vi "sv_Check Tach Info.vi"(0 "tach info":T1 {"threshold [V]" format="%.2f"}) -> (4 "avg on n pulses":i32, 6 "pulse/revolution (1)":i32, 8 "threshold":dbl format="%.2f", 10 "pulse width":i32, 15 "error code":u32)   [LabVIEW 2017]
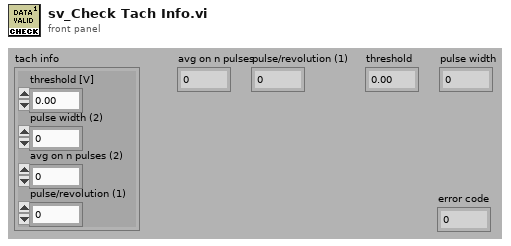
[diagram p1: front panel]
types:
  T1 = cluster{"threshold [V]":dbl, "pulse width (2)":i32, "avg on n pulses (2)":i32, "pulse/revolution (1)":i32}
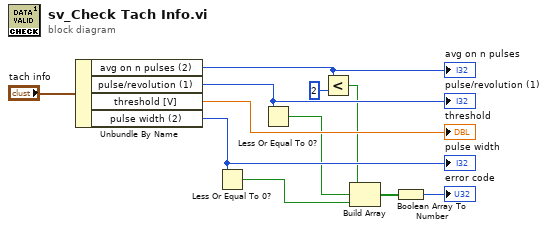
[diagram p0: block diagram]
diagram:
  n1 = Unbundle By Name("tach info") -> ("avg on n pulses (2)"=w6:i32, "pulse/revolution (1)"=w7:i32, "threshold [V]"=→"threshold":dbl, "pulse width (2)"=w10:i32)
  "pulse/revolution (1)" <- w7
  "avg on n pulses" <- w6
  "pulse width" <- w10
  n2 = Less Or Equal To 0?(x=w10) -> (x <= 0?=w3:bool)
  n3 = Less Or Equal To 0?(x=w7) -> (x <= 0?=w4:bool)
  n4 = Less?(x=w6, y=2) -> (x < y?=w5:bool)
  n5 = Build Array(w5, w4, w3) -> (w2:bool[])
  n6 = Boolean Array To Number(Boolean array=w2) -> (number=→"error code":u32)
